vi "MainUSB.vi"() -> ()   [LabVIEW 2019]
doc: "exfo test"
uses:
  <vilib>/Utility/error.llb/DialogType.ctl
  <vilib>/myRIO/Instrument Drivers/Onboard IO/UART/typedef/VISA Configuration.ctl
  <vilib>/Instr/_visa.llb/VISA Flush IO Buffer Mask.ctl
  Program Files (x86)/National Instruments/LabVIEW 2019/examples/Instrument IO/Serial/support/Serial - Settings.ctl
  <vilib>/myRIO/Instrument Drivers/Onboard IO/PWM/typedefs/PWM Reference.ctl
  <vilib>/myRIO/Common/Instrument Driver Framework/Utilities/typedefs/myRIO Generic Hardware Reference.ctl
  <vilib>/myRIO/Common/Instrument Driver Framework/Utilities/typedefs/Hardware Version Enum.ctl
  <vilib>/myRIO/Common/Instrument Driver Framework/Utilities/typedefs/myRIO v1.0 Reference.ctl
  <vilib>/myRIO/Common/Instrument Driver Framework/Utilities/typedefs/Generic FPGA Reference.ctl
  <vilib>/myRIO/Common/Instrument Driver Framework/myRIO v1.0/PWM/typedefs/PWM Channels Enum.ctl
  <vilib>/myRIO/Instrument Drivers/Onboard IO/PWM/typedefs/PWM Configuration.ctl
  <vilib>/userDefined/High Color/nirio_resource_hc.ctl
  <vilib>/myRIO/Instrument Drivers/Onboard IO/DIO/typedefs/DIO Reference.ctl
  <vilib>/myRIO/Common/Instrument Driver Framework/myRIO v1.0/DIO/typedefs/DIO Channels List.ctl
  <vilib>/myRIO/Common/Instrument Driver Framework/myRIO v1.0/DIO/typedefs/DIO Channels Enum.ctl
  <vilib>/myRIO/Instrument Drivers/Onboard IO/AO/typedefs/AO Reference.ctl
  <vilib>/myRIO/Common/Instrument Driver Framework/myRIO v1.0/AO/typedefs/AO Channels List.ctl
  <vilib>/myRIO/Common/Instrument Driver Framework/myRIO v1.0/AO/typedefs/AO Channels Enum.ctl
  <vilib>/myRIO/Common/Instrument Driver Framework/Utilities/typedefs/Analog Scaling Constants List.ctl
  <vilib>/myRIO/Common/Instrument Driver Framework/Utilities/typedefs/Analog Scaling Constants.ctl
  <vilib>/myRIO/Common/Instrument Driver Framework/Utilities/vis/Is FPGA Ref Available.vi
  <vilib>/myRIO/Common/Instrument Driver Framework/myRIO v1.0/DIO/vis/myRIO v1.1 Open DIO.vi
  <vilib>/myRIO/Instrument Drivers/Onboard IO/DIO/vis/Read.vi
  <vilib>/myRIO/Instrument Drivers/Onboard IO/DIO/vis/Write.vi
  <vilib>/myRIO/Common/Instrument Driver Framework/myRIO v1.0/PWM/vis/myRIO v1.1 Open PWM.vi
  <vilib>/myRIO/Instrument Drivers/Onboard IO/PWM/vis/Set Duty Cycle and Frequency.vi
  <vilib>/myRIO/Common/Instrument Driver Framework/myRIO v1.0/AO/vis/myRIO v1.1 Open AO.vi
  <vilib>/myRIO/Instrument Drivers/Onboard IO/AO/vis/Write.vi
  <vilib>/myRIO/Common/Instrument Driver Framework/Utilities/vis/Validate Channels.vi
  <vilib>/myRIO/Common/Instrument Driver Framework/myRIO v1.0/DIO/vis/myRIO v1.0 Reserve DIO.vi
  <vilib>/myRIO/Common/Instrument Driver Framework/myRIO v1.0/PWM/vis/myRIO v1.0 Reserve PWM.vi
  <vilib>/myRIO/Common/Instrument Driver Framework/myRIO v1.0/AO/vis/myRIO v1.0 Reserve AO.vi
  <vilib>/myRIO/Common/Instrument Driver Framework/myRIO v1.0/UART/vis/myRIO v1.0 Close UART.vi
  <vilib>/myRIO/Common/Instrument Driver Framework/myRIO v1.0/Resource Manager/vis/myRIO v1.0 Reserve Channel List.vi
  <vilib>/myRIO/Common/Instrument Driver Framework/myRIO v1.0/DIO/vis/myRIO v1.0 Build MUX Configuration DIO.vi
  <vilib>/myRIO/Common/Instrument Driver Framework/myRIO v1.0/PWM/vis/myRIO v1.0 Build MUX Configuration PWM.vi
  <vilib>/myRIO/Common/Instrument Driver Framework/myRIO v1.0/AO/vis/myRIO v1.0 Build MUX Configuration AO.vi
  <vilib>/myRIO/Common/Instrument Driver Framework/myRIO v1.0/Resource Manager/vis/myRIO v1.0 Reserve Channel.vi
  <vilib>/myRIO/Common/Instrument Driver Framework/myRIO v1.0/Resource Manager/vis/myRIO v1.0 Unreserve Channel.vi
  <vilib>/myRIO/Common/Instrument Driver Framework/myRIO v1.0/Resource Manager/vis/myRIO v1.0 Create Configuration List.vi
  <vilib>/myRIO/Common/Instrument Driver Framework/myRIO v1.0/Resource Manager/vis/myRIO v1.0 Build Mutex Name.vi
  <vilib>/Instr/_visa.llb/VISA Configure Serial Port (Serial Instr).vi
  <vilib>/Instr/_visa.llb/VISA Configure Serial Port (Instr).vi
  <vilib>/express/express shared/transition.llb/Dynamic To Waveform Array.vi
  <vilib>/express/express signal manip/GetorSetDDTAttributes/Set DDT Attributes/SetT0.vi
  <vilib>/express/express shared/transition.llb/Waveform Array To Dynamic.vi
  <vilib>/Utility/VariantDataType/GetNumericInfo.vi
  <vilib>/Utility/error.llb/Error Cluster From Error Code.vi
  <vilib>/myRIO/Common/Instrument Driver Framework/myRIO v1.0/myRIO v1.1 Open.vi
  <vilib>/myRIO/Common/Instrument Driver Framework/Utilities/vis/IO Manager.vi
  <vilib>/myRIO/Common/Instrument Driver Framework/Utilities/vis/Configuration Manager.vi
  <vilib>/myRIO/Common/Instrument Driver Framework/myRIO v1.0/Resource Manager/vis/myRIO v1.0 Configure IO.vi
  <vilib>/myRIO/Common/Instrument Driver Framework/myRIO v1.0/myRIO v1.0 Close.vi
  <vilib>/myRIO/Common/Instrument Driver Framework/myRIO v1.0/PWM/vis/myRIO v1.0 Write PWM.vi
  <vilib>/myRIO/Common/Instrument Driver Framework/myRIO v1.0/DIO/vis/myRIO v1.0 Write DIO.vi
  <vilib>/Utility/file.llb/Read Delimited Spreadsheet (DBL).vi
  <vilib>/myRIO/Common/Instrument Driver Framework/myRIO v1.0/DIO/vis/myRIO v1.0 Read DIO.vi
  <vilib>/addons/control/pid/pid.llb/PID (DBL).vi
  <vilib>/myRIO/Common/Instrument Driver Framework/myRIO v1.0/AO/vis/myRIO v1.0 Get Scaling Constants AO.vi
  <vilib>/myRIO/Common/Instrument Driver Framework/myRIO v1.0/AO/vis/myRIO v1.0 Write AO.vi
  <vilib>/myRIO/Common/Instrument Driver Framework/Utilities/vis/FPGA Ref Manager.vi
  <vilib>/myRIO/Common/Instrument Driver Framework/myRIO v1.0/myRIO v1.0 Reset FPGA.vi
  <vilib>/myRIO/Common/Instrument Driver Framework/myRIO v1.0/IRQ/vis/myRIO v1.0 IRQ Info FGV.vi
  <vilib>/myRIO/Common/Instrument Driver Framework/myRIO v1.0/IRQ/vis/myRIO v1.0 Timer IRQ Info FGV.vi
  <vilib>/myRIO/Common/Instrument Driver Framework/myRIO v1.0/IRQ/vis/myRIO v1.0 ISR Agent.vi
  <vilib>/myRIO/Instrument Drivers/Utilities/vis/Reset Index.vi
  <vilib>/myRIO/Common/Instrument Driver Framework/myRIO v1.0/Resource Manager/vis/myRIO v1.0 Block Write Resource Manager.vi
  <vilib>/express/express signal manip/GetorSetDDTAttributes/Set DDT Attributes/Set DDT Properties.xnode
  <vilib>/myRIO/Express VI/Onboard IO/PWM/PWM Express VI.xnode
  <vilib>/myRIO/Instrument Drivers/Onboard IO/PWM/vis/myRIO PWM Open.xnode
  <vilib>/myRIO/Express VI/Onboard IO/DO/DO Express VI.xnode
  <vilib>/myRIO/Instrument Drivers/Onboard IO/DIO/vis/myRIO DIO Open.xnode
  <vilib>/myRIO/Express VI/Onboard IO/DI/DI Express VI.xnode
  <vilib>/myRIO/Express VI/Onboard IO/AO/AO Express VI.xnode
  <vilib>/myRIO/Instrument Drivers/Onboard IO/AO/vis/myRIO AO Open.xnode
  <vilib>/myRIO/Instrument Drivers/Utilities/Utilities.lvlib
  <vilib>/myRIO/Instrument Drivers/Onboard IO/UART/UART.lvlib
  <vilib>/myRIO/Instrument Drivers/Onboard IO/DIO/DIO.lvlib
  <vilib>/myRIO/Instrument Drivers/Onboard IO/AO/AO.lvlib
  <vilib>/addons/control/pid/NI_PID_pid.lvlib
  <vilib>/Analysis/NI_AALBase.lvlib
  <vilib>/ptbypt/NI_PtbyPt.lvlib
  <vilib>/myRIO/Instrument Drivers/Onboard IO/PWM/PWM.lvlib
panel:
  out "speed":dbl
  in  "Duty Cycle":dbl(slide)=0.5 scale=0.36..1.0
  out "loaded":bool
  in  "Meta Load":bool caption="Manual Load"
  out "Load csv error":errorcluster
  in  "Open Button":bool
  in  "Load csv":path
  in  "Zero 2":bool
  out "Encoder Jumps":dbl(slide) scale=0.0..8.0
  in  "Scan":string(combo)="b-"
  in  "Zero":bool
  out "Laser COM Error":errorcluster
  out "tdmsfile":refnum<k34>
  out "forward":bool
  out "backward":bool
  out "Under":bool
  out "Over":bool
  out "Direction":bool=TRUE
  out "count":i32
  in  "loops":i32
  in  "high":i32=10924
  in  "low":i32=1024
  out "Loop":bool
  in  "Start Loop":bool
  out "logfile name":path
  out "USB flash drive info":string
  out "folder names":string[](array[string])
  out "filenames":string[](array[string])
  out "TDMS error":errorcluster caption="error out"
  out "Recording":bool caption="Saving Data"
  in  "Record":bool caption="Enable"
  out "?":bool
  out "?":bool
  out "Laser\nRead Errors":i32
  in  "Laser Error type of dialog":T1 items=["no dialog", "OK message", "continue or stop message", "OK message + warnings", "continue/stop + warnings"]
  out "encoder":dynamicdata(graph)
  out "Laser":dynamicdata(graph)
  out "laser":dbl
  in  "Stop":bool
  in  "Forward":bool
  in  "Reverse":bool
  out "Laser Error":bool
  in  "Load":dbl(slide) min=0.0 max=2.5 step=0.1 scale=0.0..9.0
  in  "Laser ON":bool
  out "Load":dynamicdata(graph)
  out "Load":dbl
  out "encoder":dbl
  out "Arduino \nBytes at Port":u32
  out "Laser COM exit":errorcluster
  out "Arduino Read":string
  in  "Stop":bool
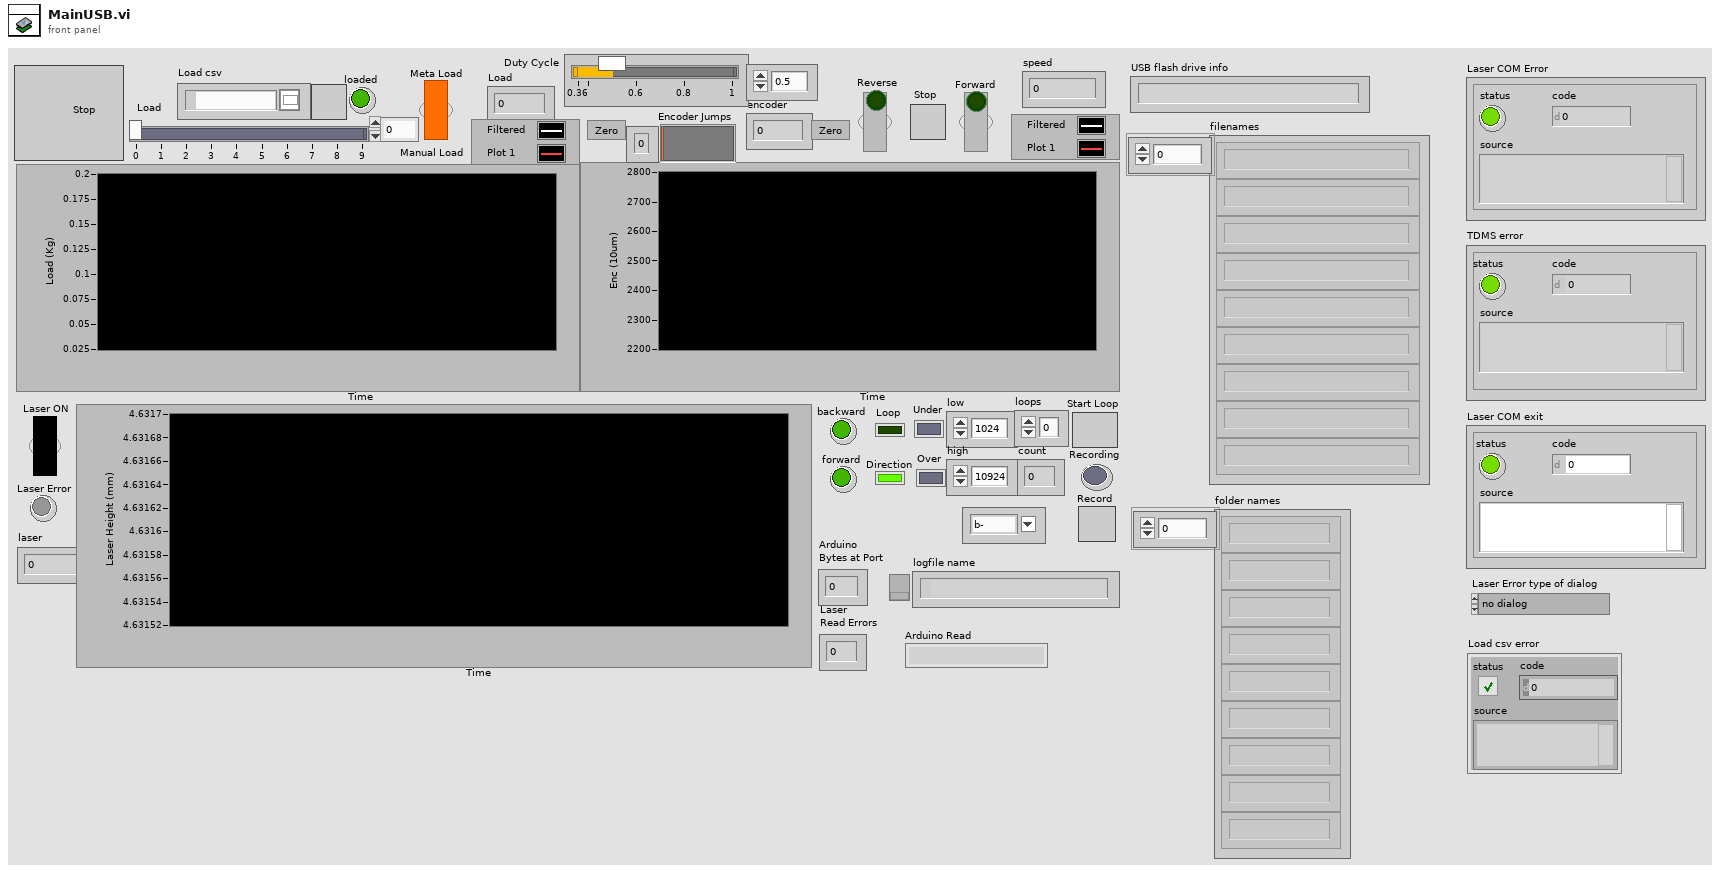
[diagram p1: front panel]
types:
  T1 = typedef "DialogType.ctl" = u16
  T2 = typedef "Serial - Settings.ctl" = cluster{"baud rate":u32, "data bits":u16, "parity":enum16{"None", "Odd", "Even", "Mark", "Space"}, "stop bits":u16, "flow control":u16}
  T3 = cluster{"proportional gain (Kc)":dbl, "integral time (Ti, min)":dbl, "derivative time (Td, min)":dbl}
  T4 = typedef "PWM.lvlib/PWM Reference.ctl" = cluster{"myRIO Reference":T5, "PWM Channels Enum":T9, "PWM Configuration":T10}
  T5 = typedef "myRIO Generic Hardware Reference.ctl" = cluster{"myRIO Model":T6, "myRIO Hardware Reference":T7}
  T6 = typedef "Hardware Version Enum.ctl" = enum16{"Unknown", "myRIO-1900", "myRIO-1950", "roboRIO", "NI ELVIS RIO CM", "ELVIS III"}
  T7 = typedef "myRIO v1.0 Reference.ctl" = cluster{"Generic FPGA Reference":T8, "Allow multiple opens":bool}
  T8 = typedef "Generic FPGA Reference.ctl" = refnum<k20>
  T9 = typedef "PWM Channels Enum.ctl" = enum16{"Not Connected", "C/PWM0", "C/PWM1", "A/PWM0", "A/PWM1", "A/PWM2", "A/PWM3", "A/PWM4", "A/PWM5", "A/PWM6", "A/PWM7", "A/PWM8", "A/PWM9", "A/PWM10", "A/PWM11", "A/PWM12", "A/PWM13", "A/PWM14", "A/PWM15", "A/PWM16", "A/PWM17", "A/PWM18", "A/PWM19", "B/PWM0", "B/PWM1", "B/PWM2", "B/PWM3", "B/PWM4", "B/PWM5", "B/PWM6", "B/PWM7", "B/PWM8", "B/PWM9", "B/PWM10", "B/PWM11", "B/PWM12", "B/PWM13", "B/PWM14", "B/PWM15", "B/PWM16", "B/PWM17", "B/PWM18", "B/PWM19", "PWM/PWM0", "PWM/PWM1", "PWM/PWM2", "PWM/PWM3", "PWM/PWM4", "PWM/PWM5", "PWM/PWM6", "PWM/PWM7", "PWM/PWM8", "PWM/PWM9"}
  T10 = typedef "PWM.lvlib/PWM Configuration.ctl" = cluster{"Frequency":dbl, "Duty Cycle":dbl}
  T11 = typedef "nirio_resource_hc.ctl" = tag
  T12 = enum16{"open", "open or create", "create or replace", "create", "open (read-only)"}
  T13 = typedef "DIO.lvlib/DIO Reference.ctl" = cluster{"myRIO Reference":T5, "DIO Channels List":T14}
  T14 = typedef "DIO Channels List.ctl" = T15[]
  T15 = typedef "DIO Channels Enum.ctl" = enum16{"Not Connected", "C/DIO0", "C/DIO1", "C/DIO2", "C/DIO3", "C/DIO4", "C/DIO5", "C/DIO6", "C/DIO7", "A/DIO0", "A/DIO1", "A/DIO2", "A/DIO3", "A/DIO4", "A/DIO5", "A/DIO6", "A/DIO7", "A/DIO8", "A/DIO9", "A/DIO10", "A/DIO11", "A/DIO12", "A/DIO13", "A/DIO14", "A/DIO15", "A/DIO16", "A/DIO17", "A/DIO18", "A/DIO19", "B/DIO0", "B/DIO1", "B/DIO2", "B/DIO3", "B/DIO4", "B/DIO5", "B/DIO6", "B/DIO7", "B/DIO8", "B/DIO9", "B/DIO10", "B/DIO11", "B/DIO12", "B/DIO13", "B/DIO14", "B/DIO15", "B/DIO16", "B/DIO17", "B/DIO18", "B/DIO19", "LED0", "LED1", "LED2", "LED3", "Button0", "DIO/DIO0", "DIO/DIO1", "DIO/DIO2", "DIO/DIO3", "DIO/DIO4", "DIO/DIO5", "DIO/DIO6", "DIO/DIO7", "DIO/DIO8", "DIO/DIO9", "SPI/CS0", "SPI/CS1", "SPI/CS2", "SPI/CS3", "LED RADIO (Green)", "LED RADIO (Red)", "LED COMM (Green)", "LED COMM (Red)", "LED MODE (Green)", "LED MODE (Red)"}
  T16 = typedef "AO.lvlib/AO Reference.ctl" = cluster{"myRIO Reference":T5, "AO Channel List":T17, "AO Scaling Constant List":T19}
  T17 = typedef "AO Channels List.ctl" = T18[]
  T18 = typedef "AO Channels Enum.ctl" = enum16{"Not Connected", "AudioOut/Left", "AudioOut/Right", "C/AO0", "C/AO1", "A/AO0", "A/AO1", "B/AO0", "B/AO1"}
  T19 = typedef "Analog Scaling Constants List.ctl" = T20[]
  T20 = typedef "Analog Scaling Constants.ctl" = cluster{"LSB Weight (Volts)":dbl, "Offset (Volts)":dbl, "Signed?":bool}
  T21 = typedef "VISA Flush IO Buffer Mask.ctl" = u16
  T22 = typedef "UART.lvlib/VISA Configuration.ctl" = cluster{"baud rate (9600)":u32, "data bits (8)":u16, "parity (0:none)":enum16{"None", "Odd", "Even", "Mark", "Space"}, "stop bits (10: 1 bit)":u16, "flow control (0:none)":u16, "termination char\n(0xA = '\\n' = LF) ":u8, "Enable Termination\nChar (T)":bool, "timeout (10sec)":u32}
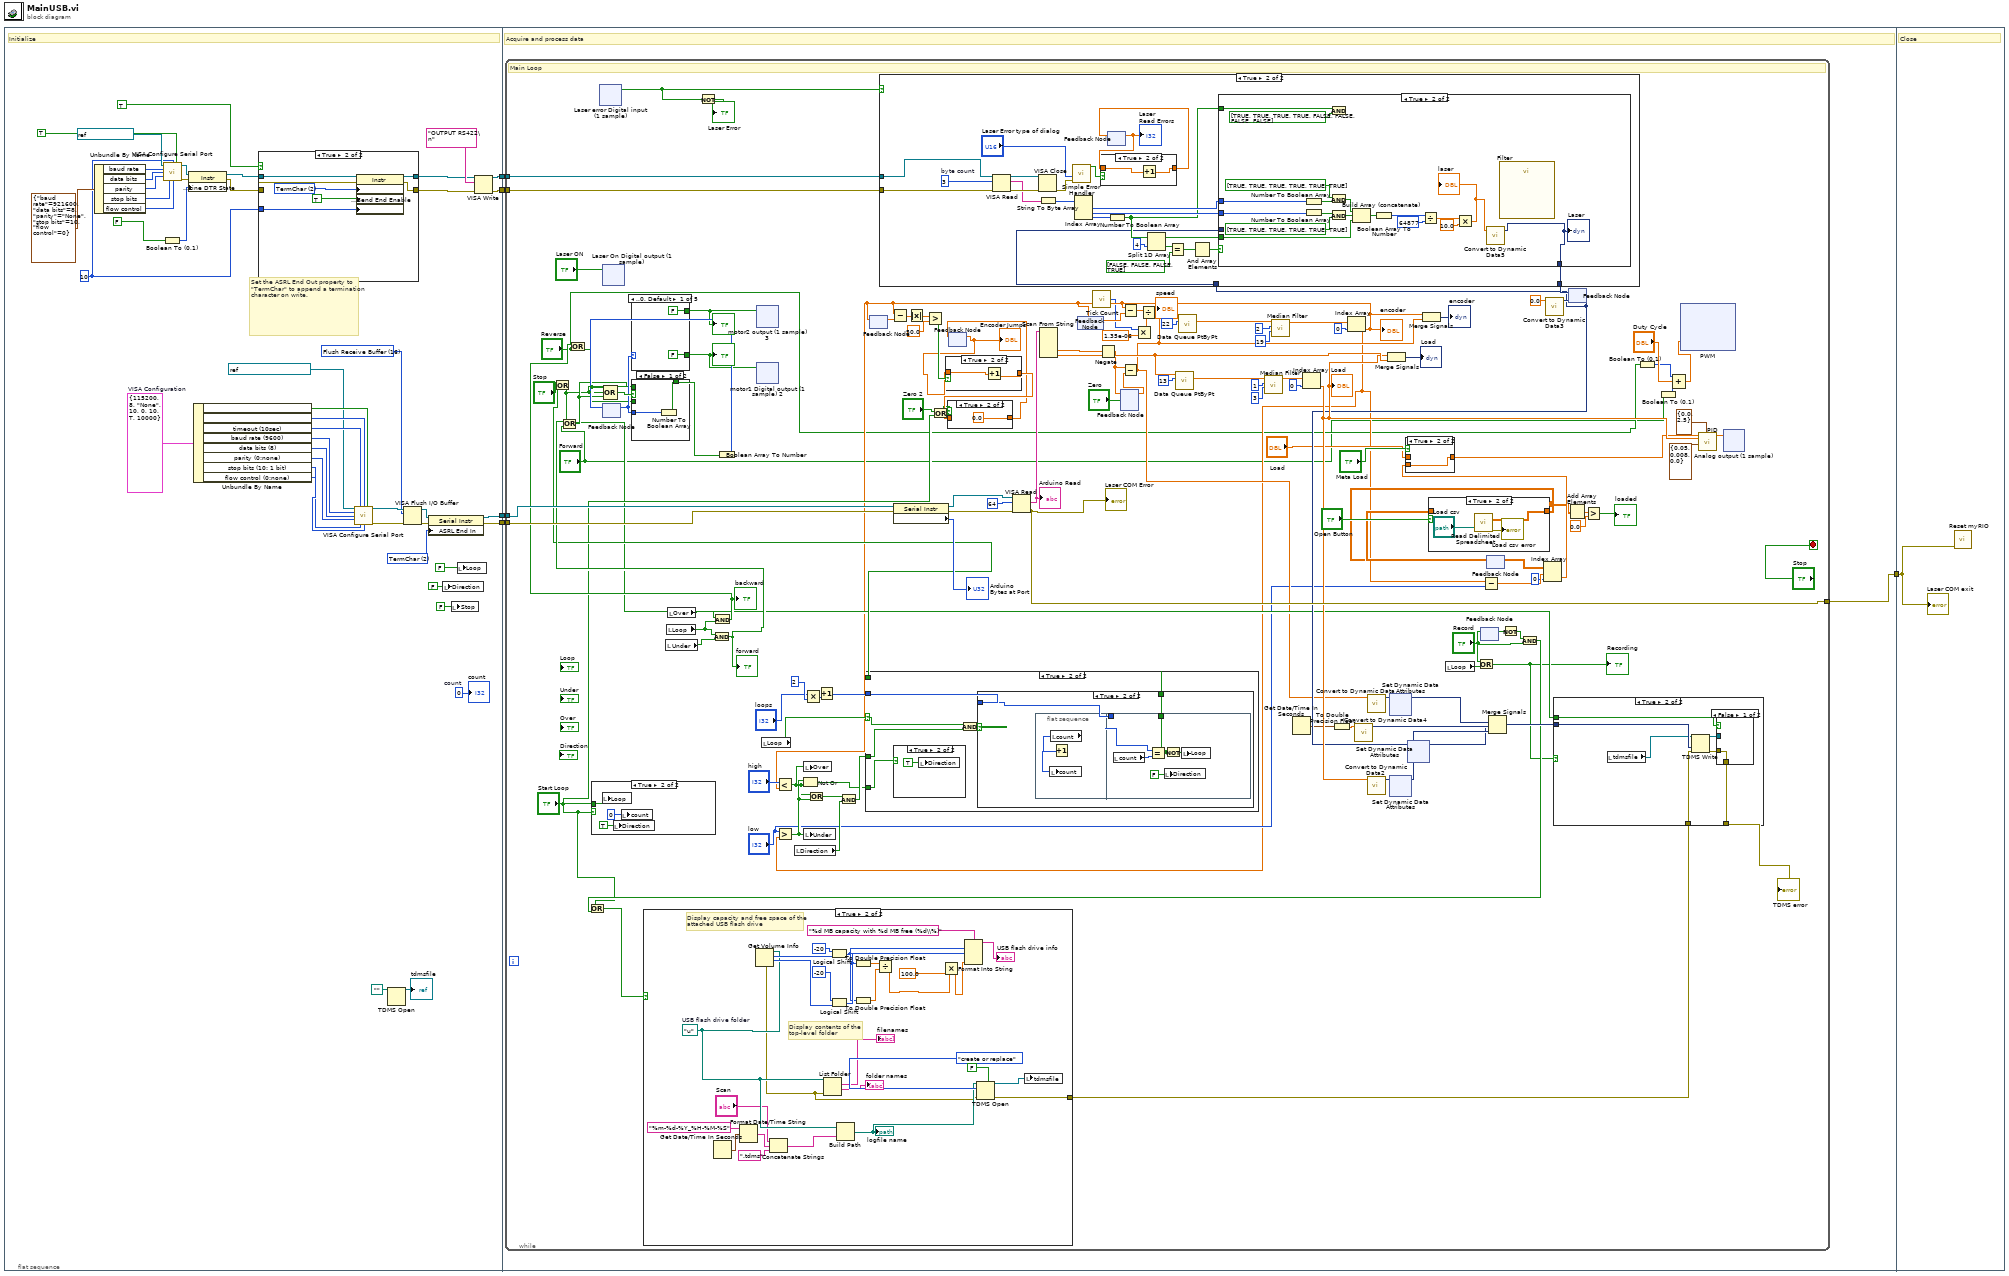
[diagram p0: block diagram]
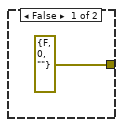
[diagram p7: hidden frame]
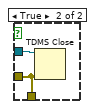
[diagram p9: hidden frame]
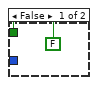
[diagram p10: hidden frame]
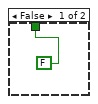
[diagram p12: hidden frame]
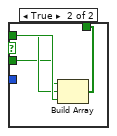
[diagram p17: hidden frame]
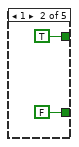
[diagram p18: hidden frame]
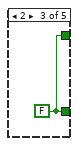
[diagram p19: hidden frame]
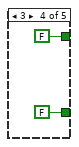
[diagram p20: hidden frame]
diagram:
  n1 = flat-sequence {
    tunnel: [w35] -> w4
    tunnel: [w34] -> w3
    tunnel: [w14] -> w2
    tunnel: [w13] -> w1
    tunnel: [w64] -> w5
    tunnel: w4 -> [w63]
    tunnel: w3 -> [w62]
    tunnel: w2 -> [w60]
    tunnel: w1 -> [w61]
    tunnel: w5 -> [w578]
    frame #0 {
      w10 = 0  # count
      w15 = u8 10 ("Termination Character")
      w11 = u16 2 items=["None", "Last Bit", "TermChar"] ("Serial Settings:End Mode for Reads")
      w38 = T21 16 items=["Flush Receive Buffer"=16, "Write Transmit Buffer to Device"=32, "Flush Receive Buffer (No I/O)"=64, "Flush Transmit Buffer"=128] ("Mask")
      w37 = T22 {"baud rate (9600)"=115200, "data bits (8)"=8, "parity (0:none)"=enum."None", "stop bits (10: 1 bit)"=10, "flow control (0:none)"=0, "termination char\n(0xA = '\\n' = LF) "=10, "Enable Termination\nChar (T)"=TRUE, "timeout (10sec)"=10000}  # VISA Configuration
      # "Set the ASRL End Out property to \"TermChar\" to append a termination character on write."
      # "Initialize"
      n2 = Unbundle By Name(T2 {"baud rate"=921600, "data bits"=8, "parity"=enum."None", "stop bits"=10, "flow control"=0} ("Serial Settings")) -> ("baud rate"=w27:u32, "data bits"=w26:u16, "parity"=w25:enum16{"None", "Odd", "Even", "Mark", "Space"}, "stop bits"=w24:u16, "flow control"=w23:u16)
      n3 = Boolean To (0,1)(Boolean=FALSE ("Assert DTR?")) -> (0, 1=w29:i16)
      n4 = call-poly "VISA Configure Serial Port"("VISA resource name"=refnum<visa-resource-name> "ASRL1::INSTR" ("VISA Refnum in"), "termination char\n(0xA = '\\n' = LF)"=w15, "Enable Termination\nChar (T)"=TRUE ("End Read on Termination Character?"), "baud rate (9600)"=w27, "data bits (8)"=w26, "parity (0:none)"=w25, "stop bits (10: 1 bit)"=w24, "flow control (0:none)"=w23) -> ("VISA resource name out"=w32:refnum<visa-resource-name>, "error out"=w31:errorcluster)  [unwired: 2 in, 4 out]
      n5 = property class="Instr"(reference=w32, error in=w31, "Serial Settings:Modem Line Settings:Line DTR State"=w29) -> (reference out=w18:refnum<visa-resource-name>, error out=w19:errorcluster)
      n6 = Unbundle By Name(w37) -> ("Enable Termination\nChar (T)"=w45:bool, "termination char\n(0xA = '\\n' = LF)"=w46:u8, "timeout (10sec)"=w44:u32, "baud rate (9600)"=w39:u32, "data bits (8)"=w40:u16, "parity (0:none)"=w41:enum16{"None", "Odd", "Even", "Mark", "Space"}, "stop bits (10: 1 bit)"=w42:u16, "flow control (0:none)"=w43:u16)
      n7 = case shown="True" TRUE ("End Write on Termination Character?") {
        tunnel: w18 -> [w51 w59]
        tunnel: w19 -> [w52 w58]
        tunnel: [w51 w57] -> w17
        tunnel: [w52 w56] -> w20
        tunnel: w15 -> [_ w54]
        frame False {
        }
        frame True {
          w55 = u16 2 items=["None", "LastBit", "TermChar", "Break"] ("Serial Settings:Serial End Mode for Writes")
          n8 = property class="Instr"(reference=w59, error in=w58, "Serial Settings:End Mode for Writes"=w55, "Message Based Settings:Send End Enable"=TRUE, "Message Based Settings:Termination Character"=w54) -> (reference out=w57:refnum<visa-resource-name>, error out=w56:errorcluster)
        }
      }
      n9 = call-poly "VISA Configure Serial Port"("VISA resource name"=refnum<visa-resource-name> "ASRL2::INSTR", "timeout (10sec)"=w44, "termination char\n(0xA = '\\n' = LF)"=w46, "Enable Termination\nChar (T)"=w45, "baud rate (9600)"=w39, "data bits (8)"=w40, "parity (0:none)"=w41, "stop bits (10: 1 bit)"=w42, "flow control (0:none)"=w43) -> ("VISA resource name out"=w48:refnum<visa-resource-name>, "error out"=w47:errorcluster)  [unwired: 5 in]
      n10 = TDMS Open(11:path "" ("file path")) -> (3:→"tdmsfile":refnum<k34>)  [unwired: 6 in, 1 out]
      n11 = VISA Flush I/O Buffer(VISA resource name=w48, mask (16)=w38, error in (no error)=w47) -> (VISA resource name out=w49:refnum<visa-resource-name>, error out=w50:errorcluster)
      n12 = property class="Serial Instr"(reference=w49, error in=w50, "ASRL End In"=w11) -> (reference out=w35:refnum<visa-resource-name>, error out=w34:errorcluster)
      n13 = local write "Direction"(FALSE ("Direction")) -> ()
      n14 = local write "Stop"(FALSE ("Stop")) -> ()
      n15 = local write "Loop"(FALSE ("Loop")) -> ()
      n16 = VISA Write(VISA resource name=w17, write buffer="OUTPUT RS422\n" ("Write String"), error in (no error)=w20) -> (VISA resource name out=w13:refnum<visa-resource-name>, error out=w14:errorcluster)  [unwired: 1 out]
      "count" <- w10
    }
    frame #1 {
      # "Acquire and process data"
      n17 = while {
        tunnel: [w187] -> w64
        tunnel: w63 -> [w186]
        tunnel: w62 -> [w185]
        tunnel: w61 -> [w155]
        tunnel: w60 -> [w154]
        stop <- "Stop" stop-if-true
        # "Main Loop"
        n18 = case shown="True" "Start Loop" {
          tunnel: "Start Loop" -> [_ w296]
          frame False {
          }
          frame True {
            n19 = local write "Loop"(w296) -> ()
            n20 = local write "Direction"(TRUE ("Direction")) -> ()
            n21 = local write "count"(0 ("count")) -> ()
          }
        }
        n22 = xnode "Laser error Digital input (1 sample)"() -> ("C/DIO1 (DIO1)"=w157:bool)  [unwired: 1 in, 1 out]
        n23 = xnode "Laser On Digital output (1 sample)"("C/DIO0 (DIO0)"="Laser ON") -> ()  [unwired: 1 in, 1 out]
        n24 = feedback #1() -> (w174:u32)  [unwired: 1 in]
        n25 = case shown="..0, Default" w174 {
          tunnel: [FALSE FALSE w466 FALSE TRUE] -> w158
          tunnel: [FALSE TRUE w466 FALSE FALSE] -> w159
          frame ..0, Default {
          }
          frame 1 {
          }
          frame 2 {
            w466 = FALSE
          }
          frame 3 {
          }
          frame 4.. {
          }
        }
        "?" <- w159
        "?" <- w158
        n26 = local read "Under"() -> (w130:bool)
        n27 = local read "Loop"() -> (w124:bool)
        n28 = local read "Over"() -> (w129:bool)
        n29 = Not(x=w157) -> (.not. x?=→"Laser Error":bool)
        n30 = And(x=w124, y=w130) -> (x .and. y?=w126:bool)
        "forward" <- w126
        n31 = Or(x=w126, y="Forward") -> (x .or. y?=w128:bool)
        n32 = And(x=w129, y=w124) -> (x .and. y?=w125:bool)
        "backward" <- w125
        n33 = Or(x=w125, y="Reverse") -> (x .or. y?=w127:bool)
        n34 = xnode "motor2 output (1 sample) 3"("C/DIO3 (DIO3)"=w159) -> ()  [unwired: 1 in, 1 out]
        n35 = xnode "motor1 Digital output (1 sample) 2"("C/DIO2 (DIO2)"=w158) -> ()  [unwired: 1 in, 1 out]
        n36 = local read "Loop"() -> (w118:bool)
        n37 = local read "Direction"() -> (w135:bool)
        n38 = Multiply(x="loops", y=2) -> (x*y=w123:i32)
        n39 = Increment(x=w123) -> (x+1=w121:i32)
        n40 = feedback #2() -> (w103:dbl)  [unwired: 1 in]
        n41 = property class="Serial Instr"(reference=w186, error in=w185) -> (reference out=w189:refnum<visa-resource-name>, error out=w182:errorcluster, "Serial Settings:Number of Bytes at Serial Port"=→"Arduino \nBytes at Port":u32)
        n42 = Or(x="Zero 2", y="Start Loop") -> (x .or. y?=w95:bool)
        n43 = feedback #3() -> (w98:dbl)  [unwired: 1 in]
        "Encoder Jumps" <- w98
        n44 = VISA Read(VISA resource name=w189, byte count=u32 64, error in (no error)=w182) -> (read buffer=w183:string, error out=w187:errorcluster)  [unwired: 2 out]
        "Arduino Read" <- w183
        "Laser COM Error" <- w187
        n45 = Scan From String(input string=w183) -> (output 2=w150:dbl, output 3=w169:dbl)  [unwired: 7 in, 3 out]
        n46 = feedback #4() -> (w77:dbl)  [unwired: 1 in]
        n47 = call "Tick Count"() -> ("Tick Count(mSec)"=w71:u32)
        n48 = Negate(x=w150) -> (-x=w107:dbl)
        n49 = feedback #5() -> (w106:dbl)  [unwired: 1 in]
        n50 = feedback-in #5(w107, "Zero") -> ()
        n51 = Subtract(x=w107, y=w106) -> (x-y=w89:dbl)
        n52 = Multiply(x=w71, y=1.35e-06) -> (x*y=w72:dbl)
        n53 = call <vilib>:"Data Queue PtByPt.vi"("sample length"=13, "input data point"=w169) -> ("Current Queue"=w172:dbl[])  [unwired: 5 in, 4 out]
        n54 = call <vilib>:"Data Queue PtByPt.vi"("sample length"=22, "input data point"=w89) -> ("Current Queue"=w164:dbl[])  [unwired: 5 in, 4 out]
        n55 = call <vilib>:"Median Filter.vi"("right rank"=3, "left rank"=1, "X"=w172) -> ("Filtered X"=w171:dbl[])  [unwired: 7 in, 1 out]
        n56 = call <vilib>:"Median Filter.vi"("right rank"=19, "left rank"=2, "X"=w164) -> ("Filtered X"=w163:dbl[])  [unwired: 7 in, 1 out]
        n57 = Get Date/Time In Seconds() -> (seconds since 1Jan1904=w141:timestamp)
        n58 = Index Array(array=w171, index=0) -> (element=w147:dbl)
        "Load" <- w147
        n59 = To Double Precision Float(number=w141) -> (double precision float=w139:dbl)
        n60 = Index Array(array=w163, index=0) -> (element=w76:dbl)
        "encoder" <- w76
        n61 = Less?(x="high", y=w76) -> (x < y?=w136:bool)
        n62 = Greater?(x="low", y=w76) -> (0:w137:bool)
        n63 = Not Or(1:w136, 2:w137) -> (0:w131:bool)
        n64 = local write "Over"(w136) -> ()
        n65 = local write "Under"(w137) -> ()
        n66 = Or(x=w136, y=w137) -> (x .or. y?=w134:bool)
        n67 = And(x=w134, y=w135) -> (x .and. y?=w132:bool)
        n68 = case shown="True" w118 {
          selector: w118 -> [_ w281]
          tunnel: w121 -> [_ w282]
          tunnel: w132 -> [_ w279]
          tunnel: w131 -> [_ w278]
          tunnel: [FALSE w277] -> w117
          frame False {
          }
          frame True {
            n69 = case shown="True" w278 {
              frame False {
              }
              frame True {
                n70 = local write "Direction"(TRUE ("Direction")) -> ()
              }
            }
            n71 = And(x=w281, y=w279) -> (x .and. y?=w280:bool)
            n72 = case shown="True" w280 {
              tunnel: w282 -> [_ w286]
              tunnel: [FALSE w285] -> w277
              frame False {
              }
              frame True {
                n73 = flat-sequence {
                  tunnel: w286 -> [w290]
                  tunnel: [w289] -> w285
                  frame #0 {
                    n74 = local read "count"() -> (w288:i32)
                    n75 = Increment(x=w288) -> (x+1=w287:i32)
                    n76 = local write "count"(w287) -> ()
                  }
                  frame #1 {
                    n77 = local read "count"() -> (w292:i32)
                    n78 = Equal?(x=w290, y=w292) -> (x = y?=w289:bool)
                    n79 = Not(x=w289) -> (.not. x?=w293:bool)
                    n80 = local write "Direction"(FALSE ("Direction")) -> ()
                    n81 = local write "Loop"(w293) -> ()
                  }
                }
              }
            }
          }
        }
        n82 = Or(x="Stop", y=w117) -> (x .or. y?=w93:bool)
        n83 = Compound Arithmetic op=OR(w127, w93, w128) -> (w178:bool)
        n84 = case shown="False" w178 {
          tunnel: w128 -> [_ w461]
          tunnel: w93 -> [_ w460]
          tunnel: w127 -> [_ w459]
          tunnel: [w456 w458] -> w176
          tunnel: w174 -> [w457 _]
          frame False {
            n85 = Number To Boolean Array(number=w457) -> (Boolean array=w456:bool[])
          }
          frame True {
            n86 = Build Array(w459, w460, w461) -> (w458:bool[])
          }
        }
        n87 = Boolean Array To Number(Boolean array=w176) -> (number=w175:u32)
        n88 = feedback-in #1(w175) -> ()
        n89 = feedback-in #2(w76) -> ()
        n90 = Subtract(x=w76, y=w103) -> (x-y=w104:dbl)
        n91 = Absolute Value(x=w104) -> (abs(x)=w102:dbl)
        n92 = Greater?(x=w102, y=50.0) -> (0:w100:bool)
        n93 = case shown="True" w100 {
          tunnel: w98 -> [w233 w235]
          tunnel: [w233 w234] -> w97
          frame False {
          }
          frame True {
            n94 = Increment(x=w235) -> (x+1=w234:dbl)
          }
        }
        n95 = case shown="True" w95 {
          tunnel: [w231 0.0] -> w96
          tunnel: w97 -> [w231 _]
          frame False {
          }
          frame True {
          }
        }
        n96 = feedback-in #3(w96) -> ()
        n97 = feedback-in #4(w76) -> ()
        n98 = Subtract(x=w76, y=w77) -> (x-y=w75:dbl)
        n99 = Divide(x=w75, y=w72) -> (x/y=→"speed":dbl)
        n100 = call "Convert to Dynamic Data4"("Double"=w139) -> ("Dynamic Data Type"=w140:dynamicdata)  [unwired: 3 in]
        n101 = call "Convert to Dynamic Data"("Double"=w89) -> ("Dynamic Data Type"=w149:dynamicdata)  [unwired: 3 in]
        n102 = call "Convert to Dynamic Data2"("Double"=w147) -> ("Dynamic Data Type"=w148:dynamicdata)  [unwired: 3 in]
        n103 = Merge Signals(w147, w169) -> (→"Load":dynamicdata)
        n104 = xnode "Set Dynamic Data Attributes"("Signals In"=w149) -> ("Signals Out"=w146:dynamicdata)  [unwired: 3 in, 1 out]
        n105 = xnode "Set Dynamic Data Attributes"("Signals In"=w148) -> ("Signals Out"=w145:dynamicdata)  [unwired: 3 in, 1 out]
        n106 = Merge Signals(w76, w89) -> (→"encoder":dynamicdata)
        n107 = local read "Loop"() -> (w138:bool)
        n108 = Or(x="Record", y=w138) -> (x .or. y?=w92:bool)
        "Recording" <- w92
        n109 = feedback-in #6("Record") -> ()
        n110 = feedback #6() -> (w112:bool)  [unwired: 1 in]
        n111 = Subtract(x=w76, y="low") -> (x-y=w87:dbl)
        n112 = feedback #7() -> (w90:dbl[][])  [unwired: 1 in]
        n113 = case shown="True" "Open Button" {
          tunnel: [w227 w229] -> w78
          tunnel: w90 -> [w227 _]
          frame False {
          }
          frame True {
            n114 = call-poly <vilib>:"Read Delimited Spreadsheet.vi"("file path (dialog if empty)"="Load csv") -> ("all rows"=w229:dbl[][], "error out"=→"Load csv error":errorcluster)  [unwired: 9 in, 4 out]
          }
        }
        n115 = feedback-in #7(w78) -> ()
        n116 = Not(x=w112) -> (.not. x?=w111:bool)
        n117 = And(x=w111, y="Record") -> (x .and. y?=w109:bool)
        n118 = Or(x="Start Loop", y=w109) -> (x .or. y?=w114:bool)
        n119 = case shown="True" w114 {
          tunnel: [errorcluster {"status"=FALSE, "code"=0, "source"=""} ("error out") w239] -> w115
          frame False {
          }
          frame True {
            w247 = path "u:/"  # USB flash drive folder
            # "Display contents of the \ntop-level folder"
            # "Display capacity and free space of the\nattached USB flash drive"
            n120 = Get Date/Time In Seconds() -> (seconds since 1Jan1904=w262:timestamp)
            n121 = Format Date/Time String(time format string (%c)="%m-%d-%Y_%H-%M-%S", seconds (now)=w262) -> (date/time string=w263:string)  [unwired: 1 in]
            n122 = Get Volume Info(11:w247) -> (0:w241:errorcluster, 1:w252:i64, 2:w253:i64)  [unwired: 1 in, 3 out]
            n123 = Concatenate Strings("Scan", w263, ".tdms" ("string")) -> (w261:string)
            n124 = List Folder(path=w247, error in=w241) -> (filenames=→"filenames":string[], folder names=→"folder names":string[])  [unwired: 2 in, 2 out]
            n125 = Logical Shift(y=i16 -20, x=w253) -> (x << y=w257:i64)
            n126 = Logical Shift(y=i16 -20, x=w252) -> (x << y=w259:i64)
            n127 = Build Path(base path=w247, name or relative path=w261) -> (appended path=w242:path)
            "logfile name" <- w242
            n128 = To Double Precision Float(number=w259) -> (double precision float=w260:dbl)
            n129 = To Double Precision Float(number=w257) -> (double precision float=w258:dbl)
            n130 = Divide(x=w260, y=w258) -> (x/y=w255:dbl)
            n131 = Multiply(x=w255, y=100.0) -> (x*y=w256:dbl)
            n132 = Format Into String "Format Into String"(format string="%d MB capacity with %d MB free (%d\\%)", w257, w259, w256) -> (resulting string=→"USB flash drive info":string)  [unwired: 2 in, 1 out]
            n133 = TDMS Open(5:FALSE ("create index file? (T)"), 8:w241, 10:T12."create or replace" ("operation"), 11:w242) -> (0:w239:errorcluster, 3:w240:refnum<k34>)  [unwired: 3 in]
            n134 = local write "tdmsfile"(w240) -> ()
          }
        }
        n135 = Index Array(array=w90, index (row)=w87, index (col)=0 ("disabled index (col)")) -> (element=w83:dbl)
        n136 = case shown="True" "Meta Load" {
          tunnel: "Load" -> [w225 _]
          tunnel: [w225 w226] -> w84
          tunnel: w83 -> [_ w226]
          frame False {
          }
          frame True {
          }
        }
        n137 = call "Convert to Dynamic Data3"("Double"=0.0) -> ("Dynamic Data Type"=w143:dynamicdata)  [unwired: 3 in]
        n138 = feedback #8(w143) -> (w142:dynamicdata)
        n139 = case shown="True" w157 {
          tunnel: w154 -> [_ w349]
          tunnel: w155 -> [_ w348]
          tunnel: [w339 w342] -> w151
          tunnel: w142 -> [w339 w341]
          frame False {
          }
          frame True {
            w347 = u32 3  # byte count
            n140 = VISA Read(VISA resource name=w348, byte count=w347, error in (no error)=w349) -> (VISA resource name out=w362:refnum<visa-resource-name>, read buffer=w344:string, error out=w363:errorcluster)  [unwired: 1 out]
            n141 = VISA Close(VISA resource name=w362, error in (no error)=w363) -> (error out=w361:errorcluster)
            n142 = String To Byte Array(string=w344) -> (unsigned byte array=w360:u8[])
            n143 = call <vilib>:"Simple Error Handler.vi"("type of dialog (OK msg:1)"="Laser Error type of dialog", "error in (no error)"=w361) -> ("error?"=w345:bool)  [unwired: 7 out]
            n144 = Index Array(array=w360) -> (element #1=w359:u8, element #2=w358:u8, element #3=w357:u8)  [unwired: 3 in]
            n145 = feedback #9() -> (w340:dbl)  [unwired: 1 in]
            "Laser\nRead Errors" <- w340
            n146 = case shown="True" w345 {
              tunnel: w340 -> [w364 w366]
              tunnel: [w364 w365] -> w343
              frame False {
              }
              frame True {
                n147 = Increment(x=w366) -> (x+1=w365:dbl)
              }
            }
            n148 = feedback-in #9(w343) -> ()
            n149 = Number To Boolean Array(number=w357) -> (Boolean array=w356:bool[])
            n150 = Split 1D Array(array=w356, index=4) -> (first subarray=w350:bool[], second subarray=w351:bool[])
            n151 = Equal?(x=w351, y=bool[] [FALSE, FALSE, FALSE, TRUE]) -> (x = y?=w352:bool[])
            n152 = And Array Elements(Boolean array=w352) -> (logical AND=w353:bool)
            n153 = case shown="True" w353 {
              tunnel: w359 -> [_ w385]
              tunnel: w358 -> [_ w383]
              tunnel: w356 -> [_ w371]
              tunnel: w350 -> [_ w370]
              tunnel: [w367 w368] -> w342
              tunnel: w341 -> [w367 _]
              frame False {
              }
              frame True {
                n154 = Number To Boolean Array(number=w385) -> (Boolean array=w372:bool[])
                n155 = Number To Boolean Array(number=w383) -> (Boolean array=w382:bool[])
                n156 = And(x=w371, y=bool[] [TRUE, TRUE, TRUE, TRUE, FALSE, FALSE, FALSE, FALSE] ("x")) -> ()  [unwired: 1 out]
                n157 = And(x=bool[] [TRUE, TRUE, TRUE, TRUE, TRUE, TRUE], y=w372) -> (x .and. y?=w373:bool[])
                n158 = And(x=w382, y=bool[] [TRUE, TRUE, TRUE, TRUE, TRUE, TRUE] ("x")) -> (x .and. y?=w374:bool[])
                n159 = Build Array (concatenate)(w373, w374, w370) -> (w379:bool[])
                n160 = Boolean Array To Number(Boolean array=w379) -> (number=w378:u32)
                n161 = Divide(x=w378, y=u32 64877) -> (x/y=w376:dbl)
                n162 = Multiply(x=w376, y=10.0) -> (x*y=w369:dbl)
                "laser" <- w369
                n163 = call "Convert to Dynamic Data5"("Double"=w369) -> ("Dynamic Data Type"=w368:dynamicdata)  [unwired: 3 in]
                "Laser" <- w368
                n164 = call "Filter"() -> ()  [unwired: 10 in, 2 out]
              }
            }
          }
        }
        n165 = xnode "Set Dynamic Data Attributes"("Signals In"=w142) -> ("Signals Out"=w116:dynamicdata)  [unwired: 3 in, 1 out]
        n166 = Merge Signals(w140, w146, w116, w145) -> (w119:dynamicdata)
        n167 = case shown="True" w92 {
          tunnel: w119 -> [_ w272]
          tunnel: w93 -> [_ w269]
          tunnel: w115 -> [w265 w268]
          tunnel: [w265 w266] -> w105
          frame False {
          }
          frame True {
            n168 = local read "tdmsfile"() -> (w267:refnum<k34>)
            n169 = TDMS Write(0:w267, 9:w272, 11:w268) -> (4:w270:refnum<k34>, 15:w271:errorcluster)  [unwired: 3 in, 2 out]
            n170 = case shown="False" w269 {
              tunnel: w271 -> [w273 w274]
              tunnel: w270 -> [_ w275]
              tunnel: [w273 w274] -> w266
              frame False {
              }
              frame True {
                n171 = TDMS Close(8:w274, 11:w275) -> ()  [unwired: 2 out]
              }
            }
          }
        }
        "TDMS error" <- w105
        n172 = feedback-in #8(w151) -> ()
        n173 = Add Array Elements(numeric array=w78) -> (sum=w81:dbl)
        n174 = Greater?(x=w81, y=0.0) -> (0:→"loaded":bool)
        n175 = Boolean To (0,1)(Boolean="Reverse") -> (0, 1=w67:i16)
        n176 = Boolean To (0,1)(Boolean="Forward") -> (0, 1=w65:i16)
        n177 = Compound Arithmetic op=ADD(w67, "Duty Cycle", w65) -> (w68:dbl)
        n178 = xnode "PWM"("Duty Cycle"=w68) -> ()  [unwired: 1 in, 1 out]
        n179 = call-poly <vilib>:"PID.vi"("output range"=cluster{"output high":dbl, "output low":dbl} {"output high"=0.0, "output low"=2.5}, "PID gains"=T3 {"proportional gain (Kc)"=0.05, "integral time (Ti, min)"=0.008, "derivative time (Td, min)"=0.0}, "process variable"=w147, "setpoint"=w84) -> ("output"=w181:dbl)  [unwired: 6 in, 1 out]
        n180 = xnode "Analog output (1 sample)"("C/AO0 (AO0)"=w181) -> ()  [unwired: 1 in, 1 out]
      }
    }
    frame #2 {
      # "Close"
      n181 = call <vilib>:"Reset myRIO.vi"("error in (no error)"=w578) -> ()  [unwired: 10 in, 1 out]
      "Laser COM exit" <- w578
    }
  }
